vi "writeSpareParts.vi"(0 "reference in":refnum<class "excelFile.lvclass">, 2 "data":string[][](array[string]), 3 "O2 exp date":string, 5 "error in (no error)":errorcluster) -> (14 "reference out":refnum<class "excelFile.lvclass">, 19 "error out":errorcluster)   [LabVIEW 2016, in "excelFile.lvclass"]
uses:
  excelFile.lvclass
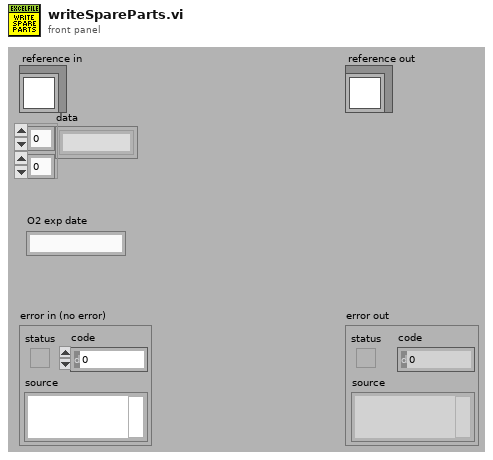
[diagram p1: front panel]
types:
  T1 = typedef "excelFile.lvclass/ObjectAttributesRef.ctl" = refnum<data-value>
  T2 = typedef "excelFile.lvclass/ObjectAttributes.ctl" = cluster{"MyAttribute":dbl, "path":string, "Refnum Excel":cluster{"Excel._Application":refnum<k7>, "Workbooks":refnum<k7>, "Open":refnum<k7>}, "data":string[][][], "save":bool, "fileType":T3, "rowsColor":u32[], "python_ref":refnum<class "python.lvclass">, "items_rows":i32[], "excel_range":i32[][], "TSR":cluster{"number":string, "TSR_path":path, "service_path":path, "email_to":string}, "excel_already_opened?":bool, "file_already_opened?":bool, "excel_protected_opened?":bool, "Refnum Cluster Worksheets":cluster{"Excel._Application":refnum<k7>, "Workbooks":refnum<k7>, "Open":refnum<k7>, "Worksheets":refnum<k7>, "Excel._Worksheet":refnum<k7>}, "#_rows_defective":i32, "#_rows_spare":i32}
  T3 = typedef "excelFile.lvclass/fileType.ctl" = enum16{"devices", "items", "partsTracking", "TSR"}
  T4 = cluster{"Excel._Application":refnum<k7>, "Workbooks":refnum<k7>, "Open":refnum<k7>, "Worksheets":refnum<k7>, "Excel._Worksheet":refnum<k7>}
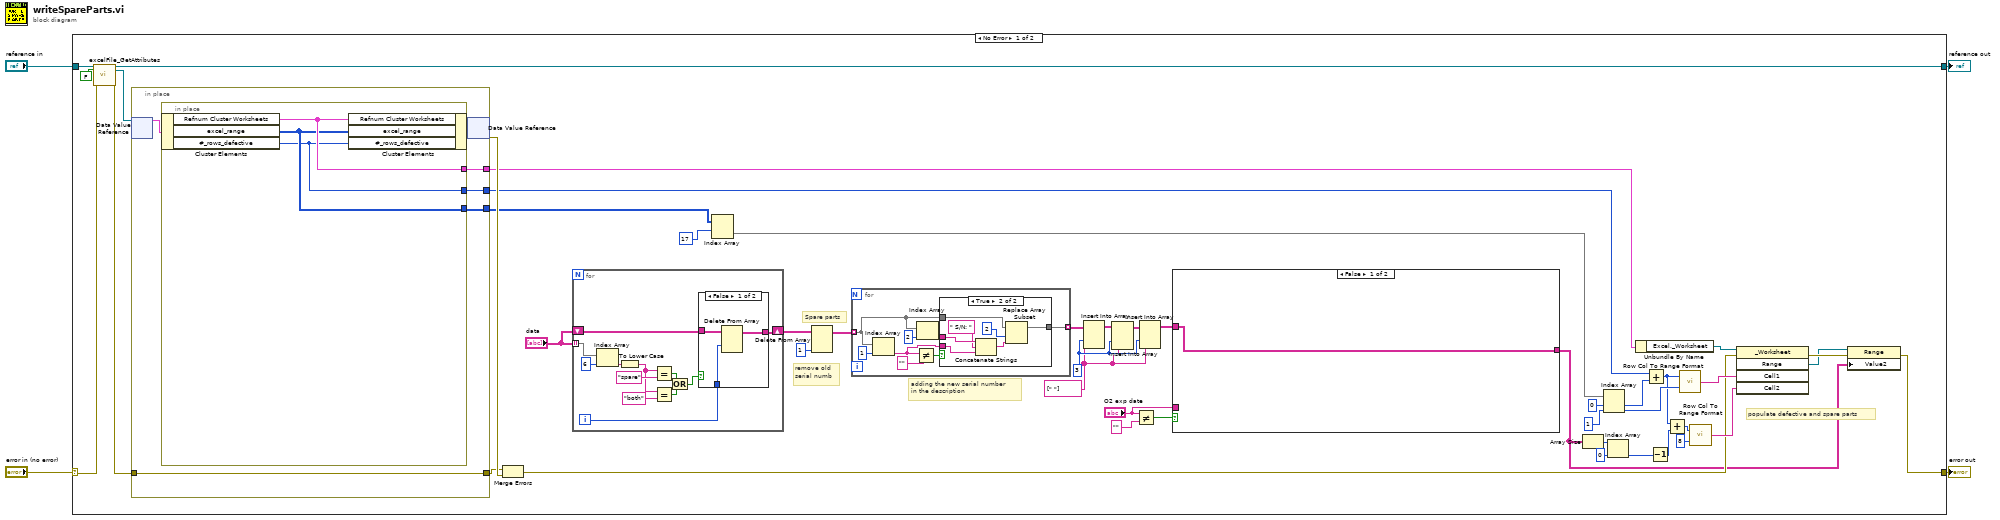
[diagram p0: block diagram]
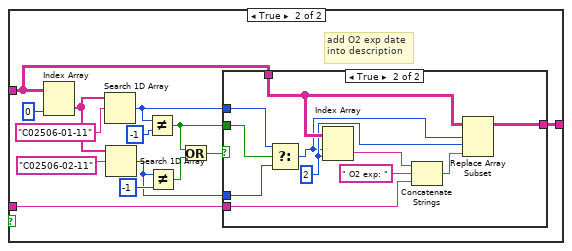
[diagram p2: hidden frame]
diagram:
  n1 = case shown="No Error" "error in (no error)" {
    selector: "error in (no error)" -> [w45 w119]
    tunnel: [w12 w119] -> w3
    tunnel: [w43 w118] -> w1
    tunnel: "reference in" -> [w47 w118]
    frame No Error {
      w17 = string[] [" "] ("new element/subarray")
      w18 = 3 ("index")
      # "adding the new serial number\nin the description"
      # "remove old\nserial numb"
      # "populate defective and spare parts"
      # "Spare parts"
      n2 = call "excelFile_GetAttributes.vi"("reference in"=w47, "return data? (T)"=FALSE, "error in (no error)"=w45) -> ("reference out"=w43:refnum<class "excelFile.lvclass">, "attributes ref"=w42:T1, "error out"=w44:errorcluster)  [unwired: 13 in, 1 out]
      n3 = in-place {
        in-place-border: w44 -> [w112]
        in-place-border: [w112] -> w48
        in-place-border: [w111] -> w15
        in-place-border: [w110] -> w40
        in-place-border: [w109] -> w10
        n4 = in-place-dvr #1(w42) -> (w113:T2)  [unwired: 1 out]
        n5 = in-place {
          in-place-border: [w117] -> w111
          in-place-border: [w116] -> w110
          in-place-border: [w115] -> w109
          n6 = in-place-cluster #2(w113) -> ("Refnum Cluster Worksheets"=w117:T4, "excel_range"=w116:i32[][], "#_rows_defective"=w115:i32)
          n7 = in-place-cluster #2("Refnum Cluster Worksheets"=w117, "excel_range"=w116, "#_rows_defective"=w115) -> (w114:T2)
        }
        n8 = in-place-dvr #1(w114) -> (w49:errorcluster)  [unwired: 1 out]
      }
      n9 = Merge Errors(w48, w49) -> (w13:errorcluster)
      n10 = for {
        tunnel: "data" -> [w104] mode=indexing
        shift-right: [w100] -> w16
        shift-left: "data" -> [w102]
        i -> [w101]
        n11 = Index Array(array=w104, index=6) -> (element=w99:string)
        n12 = To Lower Case(string=w99) -> (all lower case string=w96:string)
        n13 = Equal?(x=w96, y="both") -> (x = y?=w94:bool)
        n14 = Equal?(x=w96, y="spare") -> (x = y?=w95:bool)
        n15 = Or(x=w95, y=w94) -> (x .or. y?=w93:bool)
        n16 = case shown="False" w93 {
          tunnel: w102 -> [w107 w108]
          tunnel: w101 -> [w106 _]
          tunnel: [w105 w108] -> w100
          frame False {
            n17 = Delete From Array(array=w107, index (row)=w106) -> (array with subset deleted=w105:string[][])  [unwired: 2 in, 1 out]
          }
          frame True {
          }
        }
      }
      n18 = Index Array(array=w40, index (row)=17) -> (element=w14:i32[])  [unwired: 1 in]
      n19 = Delete From Array(array=w16, index (col)=1 ("disabled index (col)")) -> (array with subset deleted=w22:string[][])  [unwired: 2 in, 1 out]
      n20 = for {
        tunnel: w22 -> [w81] mode=indexing
        tunnel: [w78] -> w21 mode=indexing
        n21 = Index Array(array=w81, index=1) -> (element=w77:string)
        n22 = Not Equal?(x=w77, y="") -> (x != y?=w82:bool)
        n23 = Index Array(array=w81, index=2) -> (element=w79:string)
        n24 = case shown="True" w82 {
          tunnel: w81 -> [w85 w92]
          tunnel: w79 -> [_ w89]
          tunnel: [w85 w90] -> w78
          tunnel: w77 -> [_ w86]
          frame False {
          }
          frame True {
            n25 = Concatenate Strings(w89, " S/N: " ("string"), w86) -> (w88:string)
            n26 = Replace Array Subset(array=w92, new element=w88, index=2) -> (w90:string[])
          }
        }
      }
      n27 = Insert Into Array(array=w21, index (col)=w18, new element=w17) -> (w20:string[][])  [unwired: 1 in]
      n28 = Insert Into Array(array=w20, index (col)=w18, new element=w17) -> (w19:string[][])  [unwired: 1 in]
      n29 = Not Equal?(x="O2 exp date", y="") -> (x != y?=w7:bool)
      n30 = Insert Into Array(array=w19, index (col)=w18, new element=w17) -> (w9:string[][])  [unwired: 1 in]
      n31 = case shown="False" w7 {
        tunnel: w9 -> [w50 w53]
        tunnel: "O2 exp date" -> [_ w52]
        tunnel: [w50 w51] -> w5
        frame False {
        }
        frame True {
          # "add O2 exp date\ninto description"
          n32 = Index Array(array=w53, index (col)=0 ("disabled index (col)")) -> (element=w63:string[])  [unwired: 1 in]
          n33 = Search 1D Array(1D array=w63, element="C02506-01-11") -> (index of element=w55:i32)  [unwired: 1 in]
          n34 = Search 1D Array(1D array=w63, element="C02506-02-11") -> (index of element=w54:i32)  [unwired: 1 in]
          n35 = Not Equal?(x=w55, y=-1) -> (x != y?=w56:bool)
          n36 = Not Equal?(x=w54, y=-1) -> (x != y?=w58:bool)
          n37 = Or(x=w56, y=w58) -> (x .or. y?=w57:bool)
          n38 = case shown="True" w57 {
            tunnel: w56 -> [_ w76]
            tunnel: w55 -> [_ w75]
            tunnel: w54 -> [_ w74]
            tunnel: w53 -> [w65 w73]
            tunnel: w52 -> [_ w67]
            tunnel: [w65 w66] -> w51
            frame False {
            }
            frame True {
              w72 = 2 ("disabled index (col)")
              n39 = Select(t=w75, s=w76, f=w74) -> (s? t:f=w71:i32)
              n40 = Index Array(array=w73, index (row)=w71, index (col)=w72) -> (element=w69:string)
              n41 = Concatenate Strings(w69, " O2 exp: " ("string"), w67) -> (w70:string)
              n42 = Replace Array Subset(array=w73, new element=w70, index (row)=w71, index (col)=w72) -> (w66:string[][])
            }
          }
        }
      }
      n43 = Array Size(array=w5) -> (size(s)=w30:i32[])
      n44 = Index Array(array=w14, index #1=0 ("index"), index #2=1 ("index")) -> (element #1=w24:i32, element #2=w31:i32)
      n45 = Index Array(array=w30, index=0) -> (element=w26:i32)
      n46 = Unbundle By Name(w15) -> ("Excel._Worksheet"=w34:refnum<k7>)
      n47 = Add(x=w10, y=w24) -> (x+y=w11:i32)
      n48 = Decrement(x=w26) -> (x-1=w23:i32)
      n49 = Add(x=w11, y=w23) -> (x+y=w25:i32)
      n50 = call <userlib>:"Row Col To Range Format.vi"("Column"=w31, "Row"=w11) -> ("Output String"=w37:string)
      n51 = call <userlib>:"Row Col To Range Format.vi"("Column"=8, "Row"=w25) -> ("Output String"=w27:string)
      n52 = invoke class="_Worksheet" method="Range"(reference=w34, error in=w13, "Cell1"=w37, "Cell2"=w27) -> (error out=w36:errorcluster, "Range"=w35:refnum<k7>)  [unwired: 1 in, 3 out]
      n53 = property class="Range"(reference=w35, error in=w36, "Value2"=w5) -> (error out=w12:errorcluster)  [unwired: 1 out]
    }
    frame Error {
    }
  }
  "error out" <- w3
  "reference out" <- w1
